vi "sv_Insert in Swept Measurement Array.vi"(4 "read/write indices":T1(array[cluster]), 6 "AI index":i32, 7 "unscaled response magnitude":dbl format="%.2f", 8 "scaled measurements in":T2 {"harmonic components [ratio]" format="%.2f"; "THD [ratio]" format="%.2f"; "FRF Measurements"."Im [response]" format="%.2f"; "FRF Measurements"."Re [response]" format="%.2f"; "FRF Measurements"."Im [stimulus]" format="%.2f"; "FRF Measurements"."Re [stimulus]" format="%.2f"; "RMS response" format="%.2f"; "RMS stimulus" format="%.2f"}, 10 "AI freq index":i32, 11 "measurements in":T3 {"scaled response magnitude" format="%.3f"; "Harm[]" format="%.2f"; "THD" format="%.2f"; "Im [response]" format="%.2f"; "Re [response]" format="%.2f"; "Im [stimulus]" format="%.2f"; "Re [stimulus]" format="%.2f"; "RMS response" format="%.2f"; "RMS stimulus" format="%.2f"}) -> (3 "measurements out":T3 {"scaled response magnitude" format="%.3f"; "Harm[]" format="%.2f"; "THD" format="%.2f"; "Im [response]" format="%.2f"; "Re [response]" format="%.2f"; "Im [stimulus]" format="%.2f"; "Re [stimulus]" format="%.2f"; "RMS response" format="%.2f"; "RMS stimulus" format="%.2f"})   [LabVIEW 2017, in "SoundVib_SweptSine.lvlib"]
uses:
  <vilib>/addons/Sound and Vibration/svt_Swept Sine/SoundVib_SweptSine.lvlib
  <vilib>/addons/Sound and Vibration/svt_Swept Sine/subVIs/sv_Swept Sine Measurements.ctl
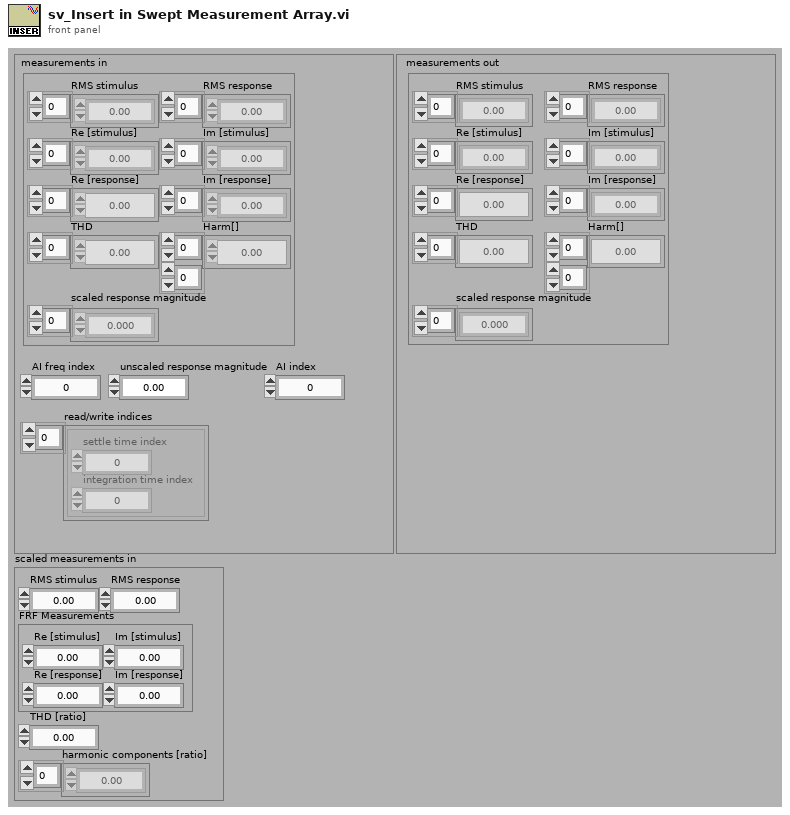
[diagram p1: front panel]
types:
  T1 = cluster{"settle time index":u32, "integration time index":u32}[]
  T2 = cluster{"RMS stimulus":dbl, "RMS response":dbl, "FRF Measurements":cluster{"Re [stimulus]":dbl, "Im [stimulus]":dbl, "Re [response]":dbl, "Im [response]":dbl}, "THD [ratio]":dbl, "harmonic components [ratio]":dbl[]}
  T3 = typedef "SoundVib_SweptSine.lvlib/sv_Swept Sine Measurements.ctl" = cluster{"RMS stimulus":dbl[], "RMS response":dbl[], "Re [stimulus]":dbl[], "Im [stimulus]":dbl[], "Re [response]":dbl[], "Im [response]":dbl[], "THD":dbl[], "Harm[]":dbl[][], "scaled response magnitude":dbl[]}
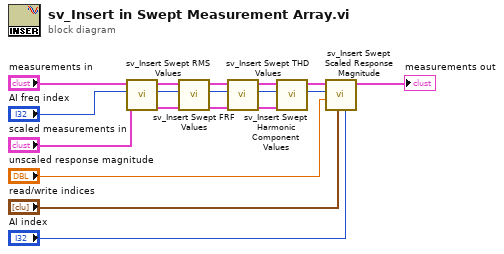
[diagram p0: block diagram]
diagram:
  n1 = call <vilib>:"sv_Insert Swept RMS Values.vi"("scaled measurements in"="scaled measurements in", "AI freq index"="AI freq index", "measurements in"="measurements in") -> ("scaled measurements in"=w17:T2, "dup AI freq index"=w8:i32, "measurements out"=w18:T3)  [unwired: 6 in]
  n2 = call <vilib>:"sv_Insert Swept FRF Values.vi"("scaled measurements in"=w17, "AI freq index"=w8, "measurements in"=w18) -> ("dup new measurements"=w16:T2, "dup AI freq index"=w6:i32, "measurements in"=w15:T3)  [unwired: 6 in]
  n3 = call <vilib>:"sv_Insert Swept THD Values.vi"("scaled measurements in"=w16, "AI freq index"=w6, "measurements in"=w15) -> ("dup new measurements"=w13:T2, "dup AI freq index"=w5:i32, "measurements out"=w14:T3)  [unwired: 6 in]
  n4 = call <vilib>:"sv_Insert Swept Harmonic Component Values.vi"("scaled measurements in"=w13, "AI freq index"=w5, "measurements in"=w14) -> ("dup AI freq index"=w4:i32, "measurements out"=w12:T3)  [unwired: 6 in, 1 out]
  n5 = call <vilib>:"sv_Insert Swept Scaled Response Magnitude.vi"("AI index"="AI index", "read/write indices"="read/write indices", "unscaled response magnitude"="unscaled response magnitude", "AI freq index"=w4, "measurements in"=w12) -> ("measurements out"=→"measurements out":T3)  [unwired: 6 in]
